vi "Read Charact Standard List.vi"(8 "error in (no error)":errorcluster, 11 "SG 18GHz Path Group in":refnum<class "SG 18GHz Path Group.lvclass">) -> (0 "error out":errorcluster, 2 "Charact Standard List":T1[](array[typedef]), 3 "SG 18GHz Path Group out":refnum<class "SG 18GHz Path Group.lvclass">)   [LabVIEW 2023, in "RFFixtureCharact.RFPM.lvlib" / "SG 18GHz Path Group.lvclass"]
uses:
  SG 18GHz Path Group.lvclass
  Instruments/Cal Standard/Type Definitions/Standard Type.ctl
  Instruments/RFFixtureCharact.Instruments.lvlib
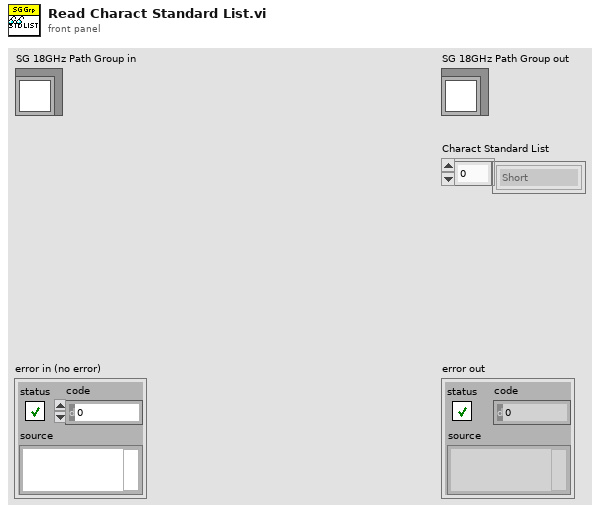
[diagram p1: front panel]
types:
  T1 = typedef "RFFixtureCharact.Instruments.lvlib/Standard Type.ctl" = enum16{"Short", "Open", "Load", "PowerMeter", "None"}
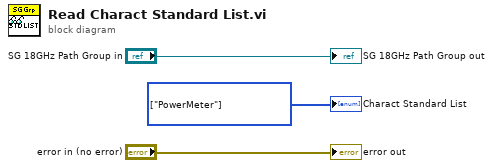
[diagram p0: block diagram]
diagram:
  w2 = T1[] [enum."PowerMeter"] items=["Short", "Open", "Load", "PowerMeter", "None"] ("Charact Standard List")
  "error out" <- "error in (no error)"
  "SG 18GHz Path Group out" <- "SG 18GHz Path Group in"
  "Charact Standard List" <- w2
